vi "Split 20  To 10.vi"(3 "IN 19:0":fxp<+,20,20> format="%08b") -> (0 "OUT 19:10":fxp<+,10,10> format="%08b", 1 "OUT 9:0":fxp<+,10,10> format="%08b")   [LabVIEW 2019]
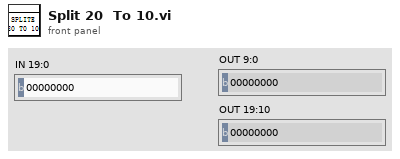
[diagram p1: front panel]
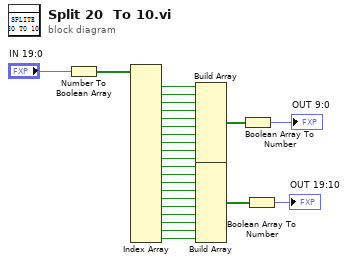
[diagram p0: block diagram]
diagram:
  n1 = Number To Boolean Array(number="IN 19:0") -> (Boolean array=w24:bool[])
  n2 = Index Array(array=w24) -> (element #1=w23:bool, element #2=w22:bool, element #3=w21:bool, element #4=w20:bool, element #5=w19:bool, element #6=w18:bool, element #7=w17:bool, element #8=w16:bool, element #9=w15:bool, element #10=w14:bool, element #11=w12:bool, element #12=w11:bool, element #13=w10:bool, element #14=w9:bool, element #15=w8:bool, element #16=w7:bool, element #17=w6:bool, element #18=w5:bool, element #19=w4:bool, element #20=w3:bool)  [unwired: 20 in]
  n3 = Build Array(w23, w22, w21, w20, w19, w18, w17, w16, w15, w14) -> (w13:bool[])
  n4 = Build Array(w12, w11, w10, w9, w8, w7, w6, w5, w4, w3) -> (w1:bool[])
  n5 = Boolean Array To Number ("布尔数组至数值转换")(Boolean array=w13) -> (number=→"OUT 9:0":fxp<+,10,10>)
  n6 = Boolean Array To Number ("布尔数组至数值转换")(Boolean array=w1) -> (number=→"OUT 19:10":fxp<+,10,10>)
